vi "user initialization.vi"(8 "error in":errorcluster, 10 "configuration in":refnum<class "control module configuration.lvclass">, 11 "fixed channel runtime in":refnum<class "GPIC Core runtime.lvclass">) -> (0 "error out":errorcluster, 3 "fixed channel runtime out":refnum<class "GPIC Core runtime.lvclass">)   [LabVIEW 2017, in "GPIC Core runtime.lvclass"]
uses:
  GPIC Core runtime.lvclass
  <vilib>/NI/DCAF/Tag Editor Core/control module/configuration/control module configuration.lvclass
  <vilib>/NI/Tag Bus Module Framework/FPGA manager/methods.ctl
  <vilib>/userdefined/High Color/nirio_resource_hc.ctl
  GPIC Core runtime.lvclass/GPIC Core runtime.ctl
  <vilib>/NI/DCAF/Tag Editor Core/control module/runtime/control module runtime.lvclass
  <vilib>/NI/Tag Bus Module Framework/FPGA manager/FPGA manager.lvlib
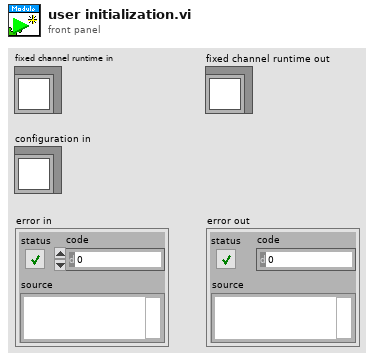
[diagram p1: front panel]
types:
  T1 = typedef "nirio_resource_hc.ctl" = tag
  T2 = typedef "FPGA manager.lvlib/methods.ctl" = enum16{"initialize bitfile", "cache bitfile", "locate bitfile", "close bitfile", "clear manager"}
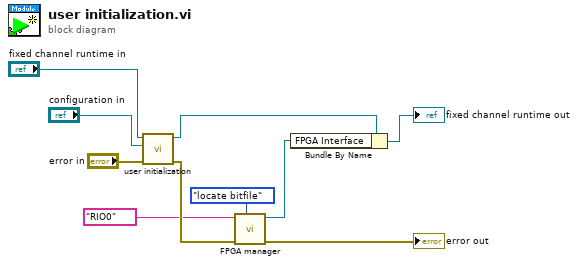
[diagram p0: block diagram]
diagram:
  n1 = call-parent "user initialization.vi"("error in"="error in", "configuration in"="configuration in", "fixed channel runtime in"="fixed channel runtime in") -> ("error out"=w6:errorcluster, "fixed channel runtime out"=w4:refnum<class "GPIC Core runtime.lvclass">)  [unwired: 7 in]
  n2 = call <vilib>:"FPGA manager.vi"("action"=methods."locate bitfile", "error in"=w6, "RIO resource"=T1 "RIO0") -> ("error out"=→"error out":errorcluster, "bitfile"=w5:refnum<k20>)  [unwired: 6 in, 1 out]
  n3 = Bundle By Name(cluster=w4, "FPGA Interface"=w5) -> (→"fixed channel runtime out":refnum<class "GPIC Core runtime.lvclass">)
